vi "Compress LIDAR Data.vi"(8 "Compression Factor":i32, 10 "Direction":dbl[](array[numeric]), 11 "Magnitude":dbl[](array[numeric])) -> (2 "Compressed Direction":dbl[](array[numeric]), 3 "Compressed Magnitude":dbl[](array[numeric]))   [LabVIEW 2018]
panel:
  # "NOTE - input directions are assumed to be sorted!"
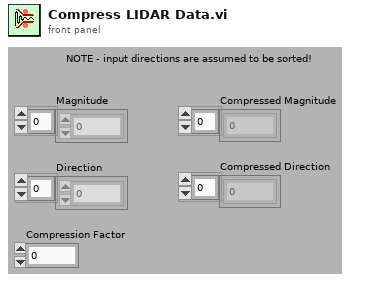
[diagram p1: front panel]
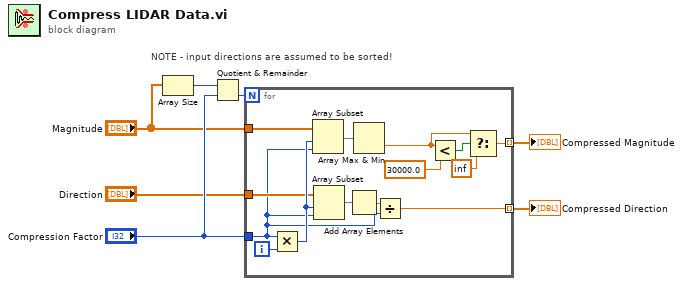
[diagram p0: block diagram]
diagram:
  # "NOTE - input directions are assumed to be sorted!"
  n1 = Array Size(array="Magnitude") -> (size(s)=w1:i32)
  n2 = Quotient & Remainder(x=w1, y="Compression Factor") -> (floor(x/y)=w2:i32)  [unwired: 1 out]
  n3 = for {
    N: w2 -> [_]
    tunnel: "Magnitude" -> [w21]
    tunnel: "Direction" -> [w18]
    tunnel: "Compression Factor" -> [w15]
    tunnel: [w11] -> w7 mode=indexing
    tunnel: [w13] -> w6 mode=indexing
    i -> [w20]
    n4 = Multiply(x=w15, y=w20) -> (x*y=w19:i32)
    n5 = Array Subset(array=w21, index=w19, length=w15) -> (w14:dbl[])
    n6 = Array Subset(array=w18, index=w19, length=w15) -> (w17:dbl[])
    n7 = Add Array Elements(numeric array=w17) -> (sum=w16:dbl)
    n8 = Array Max & Min(array=w14) -> (min value=w12:dbl)  [unwired: 3 out]
    n9 = Divide(x=w16, y=w15) -> (x/y=w13:dbl)
    n10 = Less?(x=w12, y=30000.0) -> (x < y?=w8:bool)
    n11 = Select(t=w12, s=w8, f=inf) -> (s? t:f=w11:dbl)
  }
  "Compressed Magnitude" <- w7
  "Compressed Direction" <- w6
